vi "Broadcast Exit.vi"(6 "Exit String (Exit)":string="Exit", 8 "error in":errorcluster, 10 "Message Send Parameters":variant) -> (0 "error out":errorcluster)   [LabVIEW 2013, in "Main MsgQ.lvlib"]
uses:
  Main MsgQ.lvlib
  Common/Interloop MessageQ/Message que instance modes enum.ctl
  Common/Interloop MessageQ/Interloop MessageQ.lvlib
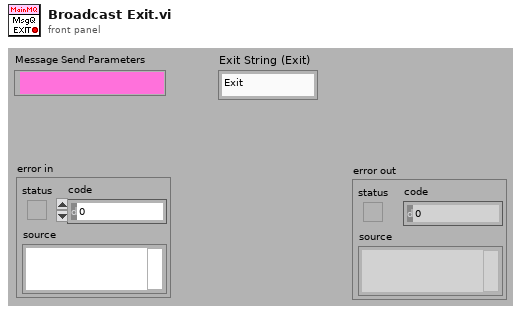
[diagram p1: front panel]
types:
  T1 = typedef "Interloop MessageQ.lvlib/Message que instance modes enum.ctl" = enum16{"Initialize", "Broadcast Message", "Send Message", "Read Message", "Kill"}
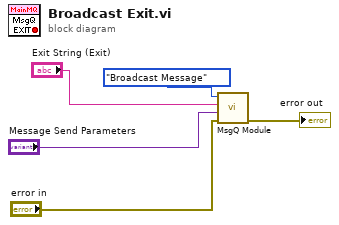
[diagram p0: block diagram]
diagram:
  n1 = call "MsgQ Module.vi"("error in (no error)"="error in", "Message Send Parameters"="Message Send Parameters", "Message Send String"="Exit String (Exit)", "Mode"=Message_que_instance_modes_enum."Broadcast Message") -> ("error out"=→"error out":errorcluster)  [unwired: 4 in, 3 out]
